vi "LCM(U64).vi"(10 "B":u64, 11 "A":u64) -> (3 "LCM":u64)   [LabVIEW 2023, in "d8.lvlib"]
uses:
  d8.lvlib
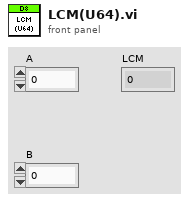
[diagram p1: front panel]
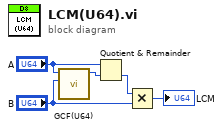
[diagram p0: block diagram]
diagram:
  n1 = call "GCF(U64).vi"("B"="B", "A"="A") -> ("GCF"=w5:u64)  [unwired: 9 in]
  n2 = Quotient & Remainder(x="A", y=w5) -> (floor(x/y)=w2:u64)  [unwired: 1 out]
  n3 = Multiply(x=w2, y="B") -> (x*y=→"LCM":u64)
